vi "niHWS Open File.vi"(8 "error in (no error)":errorcluster, 10 "permissions (0:read only)":T1, 11 "file path":path) -> (0 "error out":errorcluster, 3 "file handle":u32)   [LabVIEW 2013]
doc: "Opens or creates an HWS waveform file. The file must be closed with the niHWS Close File VI."
uses:
  niHWS Open File Permissions ID.ctl
  nihwsu.dll
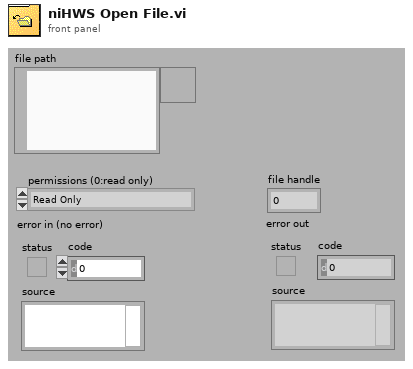
[diagram p1: front panel]
types:
  T1 = typedef "niHWS Open File Permissions ID.ctl" = enum32{"Read Only", "Read/Write Existing", "Read/Write/Create New", "Read/Write/Create New Always"}
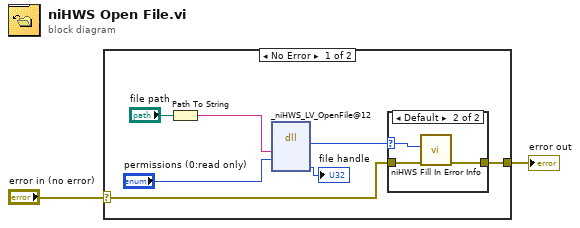
[diagram p0: block diagram]
diagram:
  n1 = case shown="No Error" "error in (no error)" {
    selector: "error in (no error)" -> [w3 w14]
    tunnel: [w6 w14] -> w1
    frame No Error {
      n2 = Path To String(path="file path") -> (string=w4:string)
      n3 = dll-call lib="nihwsu.dll" fn="_niHWS_LV_OpenFile@12"("path"=w4, "permissions"="permissions (0:read only)") -> (w5:i32, "fileHandle"=→"file handle":u32)  [unwired: 6 in, 2 out]
      n4 = case shown="Default" w5 {
        selector: w5 -> [_ w11]
        tunnel: [w10 w12] -> w6
        tunnel: w3 -> [w10 w13]
        frame 0 {
        }
        frame Default {
          n5 = call "niHWS Fill In Error Info.vi"("error in (no error)"=w13, "status code"=w11) -> ("error out"=w12:errorcluster)  [unwired: 9 in]
        }
      }
    }
    frame Error {
    }
  }
  "error out" <- w1
